vi "GetQueue.vi"() -> (0 "error out":errorcluster, 3 "Singleton Queue":refnum<queue>)   [LabVIEW 2013, in "PassDataAround.lvlib" / "PassDataAround.lvclass"]
uses:
  PassDataAround.lvclass
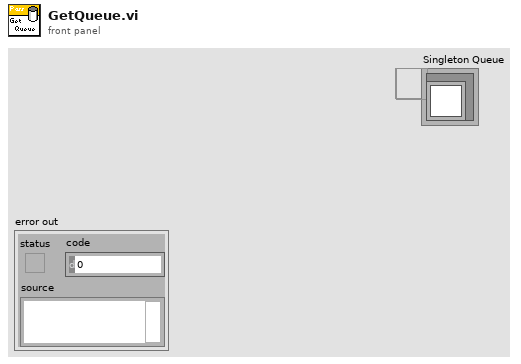
[diagram p1: front panel]
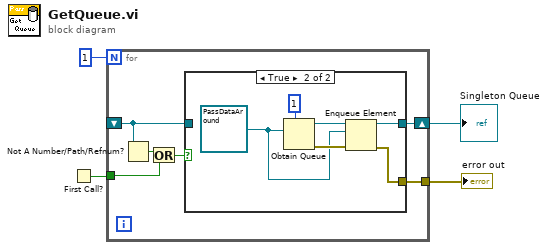
[diagram p0: block diagram]
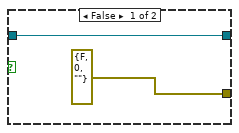
[diagram p2: hidden frame]
diagram:
  n1 = First Call?() -> (First Call?: T/F=w2:bool)
  n2 = for {
    N: 1 -> [_]
    shift-right: [w10] -> w1
    shift-left: _ -> [w8]
    tunnel: [w9] -> w3
    tunnel: w2 -> [w5]
    n3 = Not A Number/Path/Refnum?(number/path/refnum=w8) -> (NaN/Path/Refnum?=w7:bool)
    n4 = Or(x=w7, y=w5) -> (x .or. y?=w6:bool)
    n5 = case shown="True" w6 {
      tunnel: [w12 w16] -> w10
      tunnel: w8 -> [w12 _]
      tunnel: [errorcluster {"status"=FALSE, "code"=0, "source"=""} ("error out") w14] -> w9
      frame False {
      }
      frame True {
        w13 = refnum<class "PassDataAround.lvclass"> refnum ("PassDataAround.lvclass")
        n6 = Obtain Queue(max queue size (-1, unlimited)=1, element data type=w13) -> (queue out=w17:refnum<queue>, error out=w15:errorcluster)  [unwired: 3 in, 1 out]
        n7 = Enqueue Element(queue=w17, element=w13, error in (no error)=w15) -> (queue out=w16:refnum<queue>, error out=w14:errorcluster)  [unwired: 1 in, 1 out]
      }
    }
  }
  "error out" <- w3
  "Singleton Queue" <- w1
